vi "MLin-Skew-头缺分析1.vi"() -> ()   [LabVIEW 2018]
uses:
  <vilib>/vision/Measure.llb/Edge Options.ctl
  <vilib>/vision/Measure.llb/Edge Polarity.ctl
  <vilib>/vision/Contour.llb/IMAQ Contour Curve Extraction.ctl
  <vilib>/vision/Image Controls.llb/IMAQ Image.ctl
  <vilib>/vision/NI_Vision_Development_Module.lvlib
  <vilib>/vision/Contour.llb/IMAQ Connect Range Setting.ctl
panel:
  out "ImgOut":T1
  out "顶洞圆半径OK":bool
  out "error out 2":errorcluster caption="error out"
  in  "ImageSrc":T1
  in  "某偏移量":dbl format="%#_13g"
  in  "产品轴向角度":dbl
  in  "ImageDst":T1
  out "Fitted Circle":T2 {"Average SNR (dB)" format="%.2f"; "Average Strength" format="%.2f"; "Roundness (Real-World)" format="%.2f"; "Radius (Real-World)" format="%.2f"; "Center (Real-World)"."Y" format="%.2f"; "Center (Real-World)"."X" format="%.2f"; "Radius (Pixels)" format="%.2f"; "Center (Pixels)"."Y" format="%.2f"; "Center (Pixels)"."X" format="%.2f"}
  in  "顶洞圆半径上限":dbl=330.0
  in  "顶洞圆半径下限":dbl=50.0
  out "顶洞圆半径":dbl
  out "顶洞圆半径正常":bool
  out "Curvature Profile":dbl[](graph)
  in  "Curve Extraction Settings":T3={"Extraction Mode"=0, "Edge Threshold"=30, "Edge Filter Size"=2, "Min Length"=10, "Search Step Size"=10, "Max Endpoint Gap"=20, "Subpixel"=TRUE} {"Extraction Mode" items=["Normal", "Uniform Regions"]; "Edge Filter Size" items=["Fine", "Normal", "Contour Tracing"]; "Max Endpoint Gap" min=0; "Search Step Size" min=1 max=255 step=1; "Min Length" min=0; "Edge Threshold" min=1 max=350 step=1}
  in  "Kernel Width":u32=31
  in  "Contour Points Settings":T4={"Overlay?"=TRUE, "Color"=16738816, "Width"=1, "Maintain Width?"=TRUE}
  in  "顶洞_Options":T7={"Search  Direction"=0, "Edge Options"={"Edge Polarity"=0, "Kernel Size"=3, "Width"=9, "Minimum Edge Strength"=50.0, "Interpolation Type"=enum."Bilinear Fixed", "Data Processing Method"=enum."Average"}, "Show Search Area"=TRUE, "Show Search Lines"=FALSE, "Show Edges Found"=FALSE, "Show Result"=TRUE, "Search Area Color"=65280, "Search Lines Color"=255, "Edge Locations Color"=16776960, "Result Color"=16711680, "Overlay Group Name"=""} {"Search  Direction" items=["Outside to Inside", "Inside to Outside"]; "Edge Options"."Edge Polarity" items=["All Edges", "Rising Edges", "Falling Edges"]; "Edge Options"."Minimum Edge Strength" format="%.2f"; "Edge Options"."Width" step=2; "Edge Options"."Kernel Size" step=2}
  in  "顶洞_Circle Fit Options":T8={"Process"=enum."Get First Edge", "Step Size"=3.0, "Max Pixel Radius"=3}
  in  "ROI_顶洞检测扇形半张角":dbl=17.0 format="%#_13g"
  in  "R_顶洞检测小圆半径":i32=136
  in  "偏移_顶洞_向上部修正量":dbl=230.0 format="%#_13g"
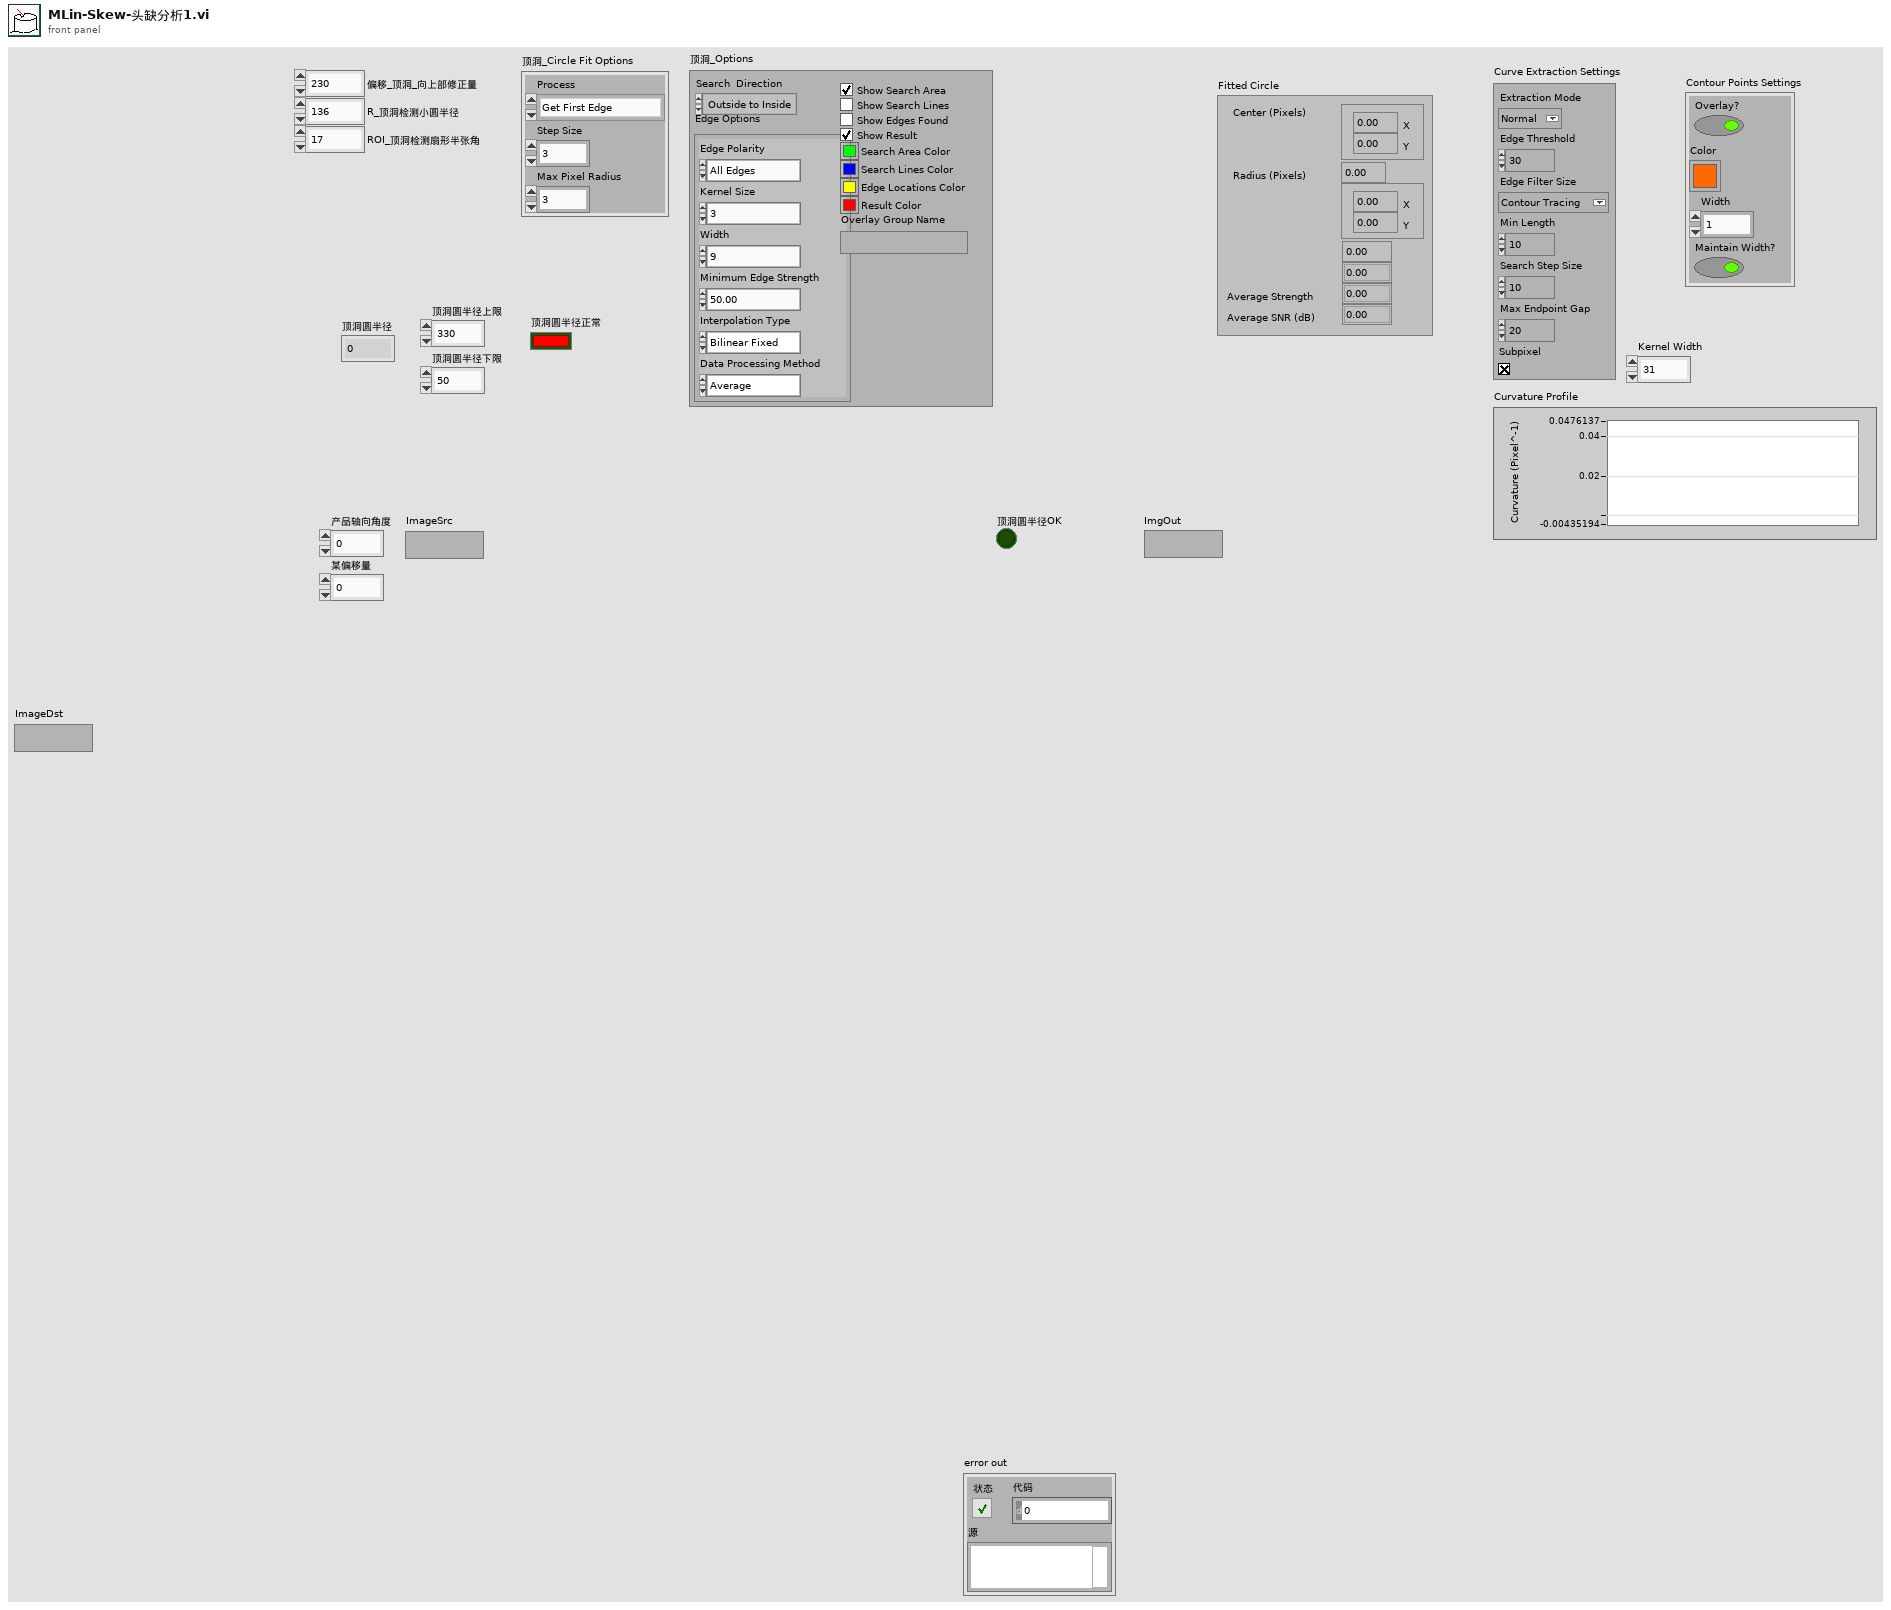
[diagram p1: front panel]
types:
  T1 = typedef "IMAQ Image.ctl" = refnum<image>
  T2 = cluster{"Center (Pixels)":cluster{"X":sgl, "Y":sgl}, "Radius (Pixels)":dbl, "Center (Real-World)":cluster{"X":sgl, "Y":sgl}, "Radius (Real-World)":dbl, "Roundness (Real-World)":dbl, "Average Strength":dbl, "Average SNR (dB)":dbl}
  T3 = typedef "IMAQ Contour Curve Extraction.ctl" = cluster{"Extraction Mode":u32, "Edge Threshold":i32, "Edge Filter Size":u32, "Min Length":i32, "Search Step Size":i32, "Max Endpoint Gap":i32, "Subpixel":bool}
  T4 = cluster{"Overlay?":bool, "Color":u32, "Width":u32, "Maintain Width?":bool}
  T5 = typedef "Edge Options.ctl" = cluster{"Edge Polarity":T6, "Kernel Size":u32, "Width":u32, "Minimum Edge Strength":sgl, "Interpolation Type":enum32{"Zero Order", "Bilinear", "Quadratic", "Cubic", "Bilinear Fixed"}, "Data Processing Method":enum32{"Average", "Median"}}
  T6 = typedef "Edge Polarity.ctl" = u32
  T7 = cluster{"Search  Direction":u32, "Edge Options":T5, "Show Search Area":bool, "Show Search Lines":bool, "Show Edges Found":bool, "Show Result":bool, "Search Area Color":u32, "Search Lines Color":u32, "Edge Locations Color":u32, "Result Color":u32, "Overlay Group Name":string}
  T8 = cluster{"Process":enum16{"Get First Edge", "Get First + Last Edge", "Get All Edges", "Get Best Edge"}, "Step Size":dbl, "Max Pixel Radius":i32}
  T9 = typedef "ROI Descriptor" = cluster{"Global Rectangle":i32[], "Contours":cluster{"ID":enum32{"External", "Internal"}, "Type":u32, "Coordinates":i32[]}[]}
  T10 = typedef "IMAQ Circle" = cluster{"Center X":i32, "Center Y":i32, "Inner Radius":i32, "Outer Radius":i32, "Start Angle":dbl, "End Angle":dbl}
  T11 = typedef "IMAQ Connect Range Setting.ctl" = cluster{"Match Constraints":u32, "Min":dbl, "Max":dbl}
  T12 = enum16{"Closest To Search Start", "Maximum Length", "Strongest Mean Gradient Change"}
  T13 = enum16{"Rect Left To Right", "Rect Right To Left", "Rect Top To Bottom", "Rect Bottom To Top", "Annulus Inner To Outer", "Annulus Outer To Inner", "Annulus Start Angle To End Angle", "Annulus End Angle To Start Angle"}
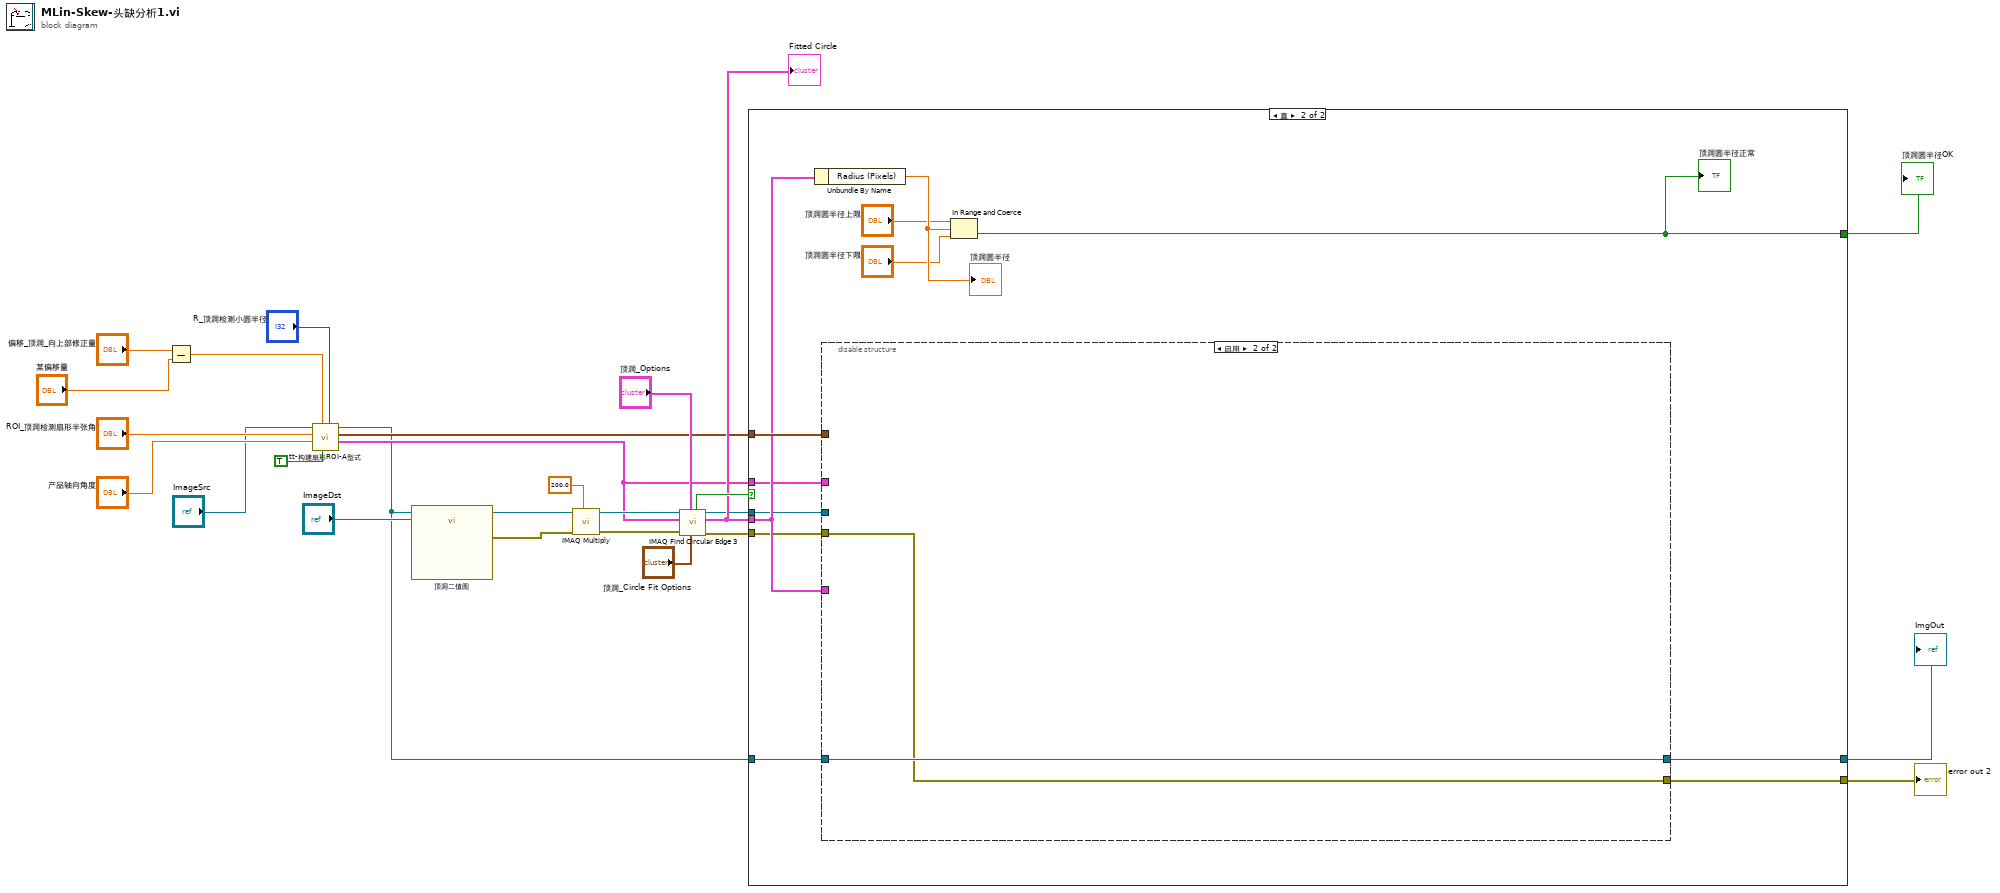
[diagram p0: block diagram]
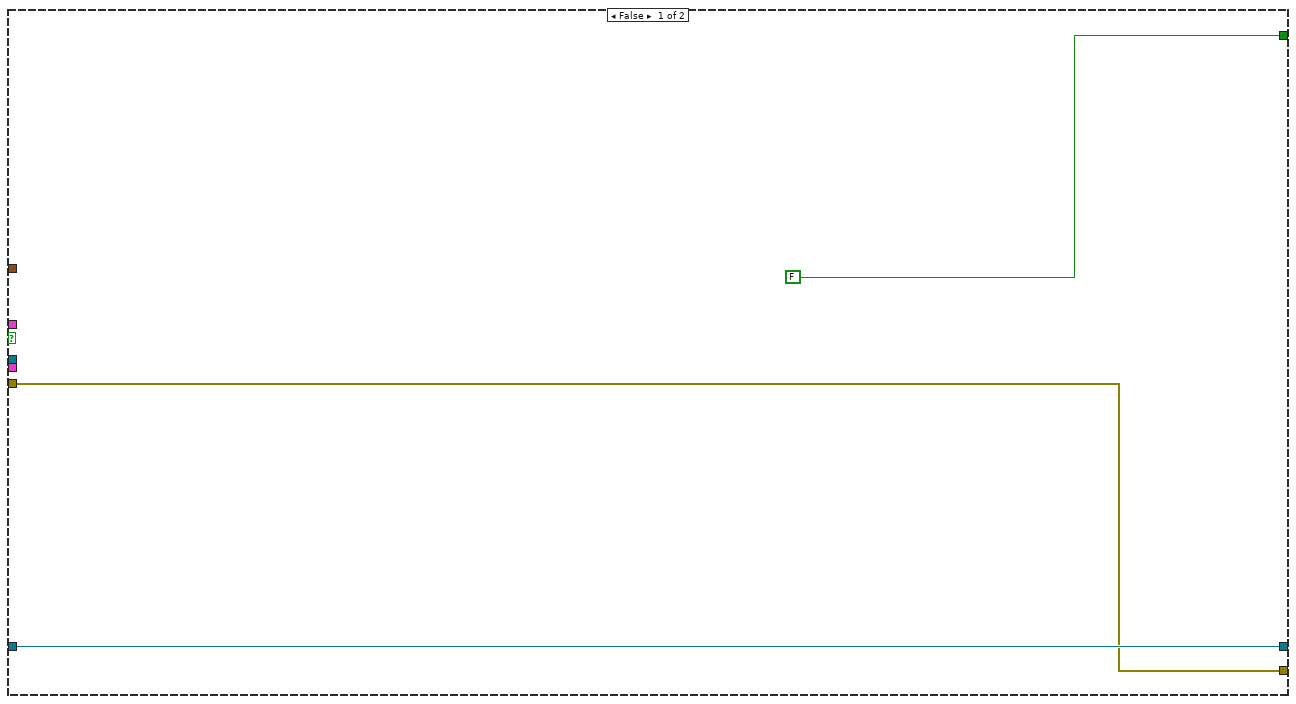
[diagram p2: hidden frame]
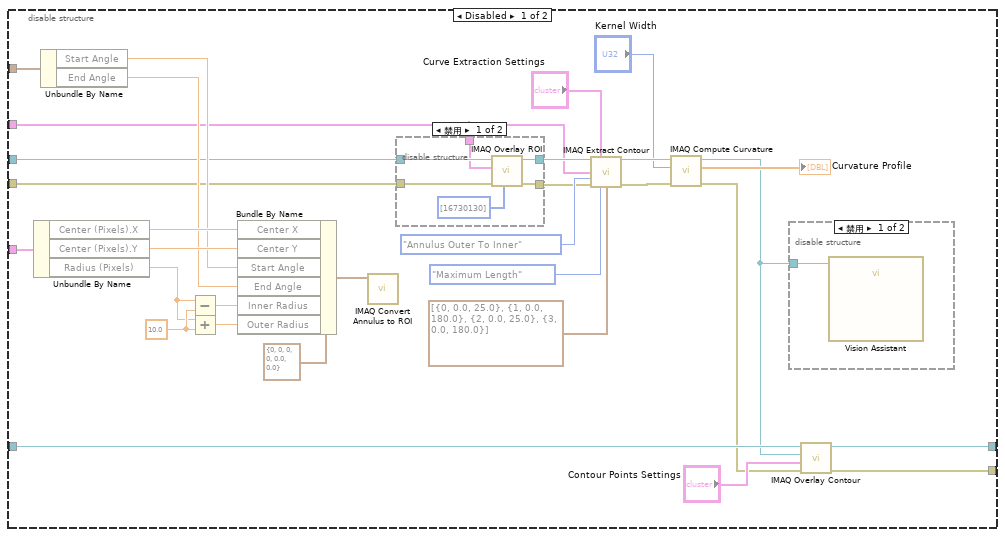
[diagram p3: hidden frame]
diagram:
  n1 = Subtract ("扣除截取半径与实际半径的差异")(x="偏移_顶洞_向上部修正量", y="某偏移量") -> (x-y=w24:dbl)
  n2 = call "tt-构建扇形ROI-A型式.vi"("R_ROI小圆半径"="R_顶洞检测小圆半径", "开启调试显示"=TRUE, "钩端向上部偏移量"=w24, "镜像产品角度"="产品轴向角度", "扇形半张角"="ROI_顶洞检测扇形半张角", "ImageSrc"="ImageSrc") -> ("anROI"=w7:T9, "输出RECT"=w10:T10, "ImgOut"=w1:T1)  [unwired: 2 in, 1 out]
  n3 = call "顶洞二值图"("Image In"=w1, "Image Dst"="ImageDst") -> ("Image Out"=w21:T1, "error out"=w20:errorcluster)  [unwired: 24 in]
  n4 = call "IMAQ Multiply"("Image Src A"=w21, "Constant"=200.0, "error in (no error)"=w20) -> ("Image Dst Out"=w18:T1, "error out"=w17:errorcluster)  [unwired: 4 in]
  n5 = call "IMAQ Find Circular Edge 3"("Circle Fit Options"="顶洞_Circle Fit Options", "Options"="顶洞_Options", "error in (no error)"=w17, "ROI Descriptor"=w7, "Image"=w18) -> ("error out"=w11:errorcluster, "Fitted Circle"=w13:T2, "Image Out"=w12:T1, "Circle Found"=w14:bool)  [unwired: 2 in, 1 out]
  "Fitted Circle" <- w13
  n6 = case shown="真" w14 {
    tunnel: w13 -> [_ w36]
    tunnel: w12 -> [_ w33]
    tunnel: w11 -> [w27 w32]
    tunnel: w10 -> [_ w37]
    tunnel: [FALSE w38] -> w9
    tunnel: w1 -> [w28 w35]
    tunnel: [w28 w34] -> w8
    tunnel: w7 -> [_ w31]
    tunnel: [w27 w30] -> w6
    frame False {
    }
    frame True {
      n7 = Unbundle By Name(w36) -> ("Radius (Pixels)"=w41:dbl)
      "顶洞圆半径" <- w41
      n8 = disable-structure shown="启用" {
        disable-tunnel: w37 -> [w65 _]
        disable-tunnel: w36 -> [w64 _]
        disable-tunnel: w35 -> [w61 w83]
        disable-tunnel: [w60 w83] -> w34
        disable-tunnel: w33 -> [w49 _]
        disable-tunnel: w32 -> [w48 w82]
        disable-tunnel: w31 -> [w45 _]
        disable-tunnel: [w42 w82] -> w30
        frame Disabled {
          w71 = 10.0 ("y")
          n9 = Unbundle By Name(w64) -> ("Center (Pixels).X"=w66:sgl, "Center (Pixels).Y"=w67:sgl, "Radius (Pixels)"=w70:dbl)
          n10 = Unbundle By Name(w65) -> ("Start Angle"=w62:dbl, "End Angle"=w63:dbl)
          n11 = Subtract(x=w70, y=w71) -> (x-y=w69:dbl)
          n12 = Add(x=w70, y=w71) -> (x+y=w68:dbl)
          n13 = Bundle By Name(cluster=T10 {"Center X"=0, "Center Y"=0, "Inner Radius"=0, "Outer Radius"=0, "Start Angle"=0.0, "End Angle"=0.0} ("输出簇"), "Center X"=w66, "Center Y"=w67, "Start Angle"=w62, "End Angle"=w63, "Inner Radius"=w69, "Outer Radius"=w68) -> (w72:T10)
          n14 = call "IMAQ Convert Annulus to ROI"("Annulus"=w72) -> ()  [unwired: 8 in, 2 out]
          n15 = disable-structure shown="禁用" {
            disable-tunnel: w49 -> [w79 w81]
            disable-tunnel: w48 -> [w78 w80]
            disable-tunnel: [w77 w81] -> w47
            disable-tunnel: [w76 w80] -> w46
            disable-tunnel: w45 -> [w74 _]
            frame Disabled {
              n16 = call "IMAQ Overlay ROI"("Colors (Green)"=u32[] [16730130], "error in (no error)"=w78, "ROI Descriptor"=w74, "Image"=w79) -> ("error out"=w76:errorcluster, "Image Out"=w77:T1)  [unwired: 6 in]
            }
            frame Enabled {
            }
          }
          n17 = call "IMAQ Extract Contour"("Source Image"=w47, "Curve Extraction"="Curve Extraction Settings", "ROI Descriptor"=w45, "Search Direction"=T13."Annulus Outer To Inner", "error in (no error)"=w46, "Contour Selection"=T12."Maximum Length", "Curve Connection"=T11[] [{"Match Constraints"=0, "Min"=0.0, "Max"=25.0}, {"Match Constraints"=1, "Min"=0.0, "Max"=180.0}, {"Match Constraints"=2, "Min"=0.0, "Max"=25.0}, {"Match Constraints"=3, "Min"=0.0, "Max"=180.0}]) -> ("Source Image Out"=w58:T1, "error out"=w56:errorcluster)  [unwired: 1 in, 6 out]
          n18 = call "IMAQ Compute Curvature"("error in (no error)"=w56, "Kernel Width"="Kernel Width", "Contour Image"=w58) -> ("error out"=w43:errorcluster, "Curvature Profile (pixel)"=→"Curvature Profile":dbl[], "Contour Image Out (dup)"=w44:T1)  [unwired: 6 out]
          n19 = disable-structure shown="禁用" {
            disable-tunnel: w44 -> [w73 _]
            frame Disabled {
              n20 = call "Vision Assistant"("Image In"=w73) -> ()  [unwired: 25 in, 2 out]
            }
            frame Enabled {
            }
          }
          n21 = call "IMAQ Overlay Contour"("error in (no error)"=w43, "Contour Points Settings"="Contour Points Settings", "Contour Image"=w44, "Image"=w61) -> ("error out"=w42:errorcluster, "Image Out"=w60:T1)  [unwired: 2 in, 4 out]
        }
        frame Enabled {
        }
      }
      n22 = In Range and Coerce(upper limit="顶洞圆半径上限", x=w41, lower limit="顶洞圆半径下限") -> (In Range?=w38:bool)  [unwired: 1 out]
      "顶洞圆半径正常" <- w38
    }
  }
  "error out 2" <- w6
  "顶洞圆半径OK" <- w9
  "ImgOut" <- w8
